vi "Checksum.vi"(0 "VISA resource name":refnum<visa-resource-name>, 5 "Command Frame Array":i16[](array[numeric]), 11 "error in (no error)":errorcluster) -> (4 "VISA resource name out":refnum<visa-resource-name>, 6 "Output String":string, 8 "Output Array":i16[](array[numeric]), 10 "Checksum":i16, 15 "error out":errorcluster)   [LabVIEW 2019, in "BK Precision 178XB Series.lvlib"]
doc: "This SubVI calculates the checksum of all bytes in the <b>Command frame array</b>, which is an array of 26 bytes. The checksum value takes the sum of the first 25 bytes in the array, and places the result into the last byte (26th byte). The <b>Output array</b> will be the resulting 26 byte array with the checksum value as the element of the last byte. <b>Output string</b> is the converted string from <b>Output array</b>.\n\nThe <b>Checksum</b> output will give the value of the checksum only."
uses:
  BK Precision 178XB Series.lvlib
panel:
  # "(c) 2009 B&K PRECISION CORPORATION.  ALL RIGHTS RESERVED."
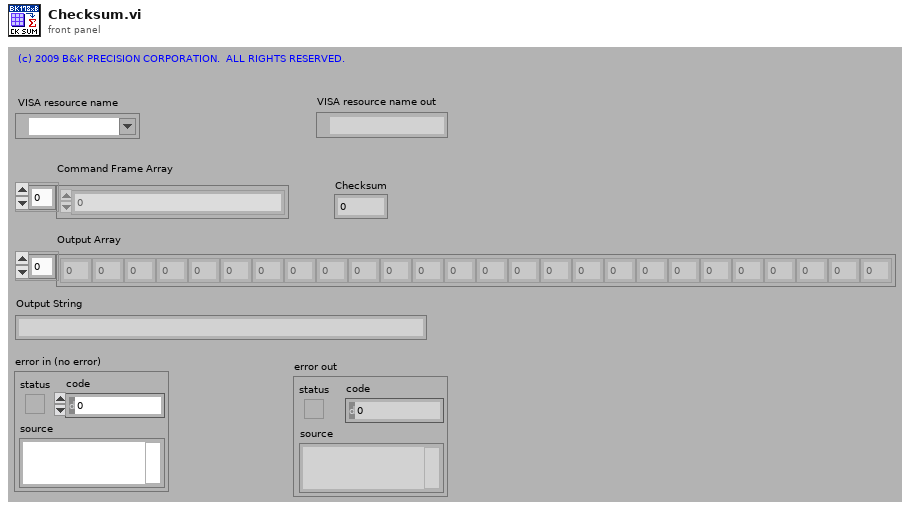
[diagram p1: front panel]
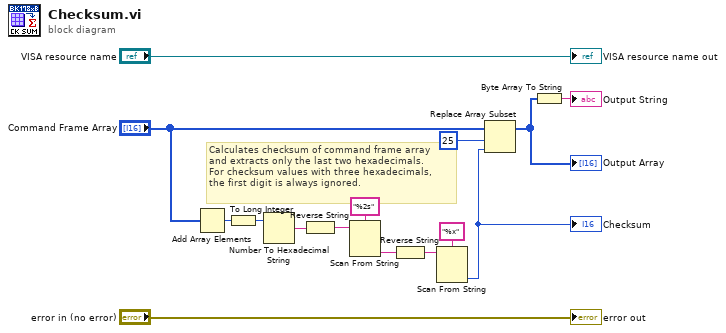
[diagram p0: block diagram]
diagram:
  # "Calculates checksum of command frame array\nand extracts only the last two hexadecimals. \nFor checksum values with three hexadecimals,\nthe first digit is always ignored."
  n1 = Add Array Elements(numeric array="Command Frame Array") -> (sum=w12:i16)
  n2 = To Long Integer(number=w12) -> (32bit integer=w14:i32)
  n3 = Number To Hexadecimal String(2:w14) -> (0:w8:string)  [unwired: 1 in]
  n4 = Reverse String(1:w8) -> (0:w15:string)
  n5 = Scan From String(format string="%2s", input string=w15) -> (output 1=w11:string)  [unwired: 3 in, 3 out]
  n6 = Reverse String(1:w11) -> (0:w10:string)
  n7 = Scan From String(format string="%x", input string=w10) -> (output 1=w4:i16)  [unwired: 3 in, 3 out]
  "Checksum" <- w4
  n8 = Replace Array Subset(array="Command Frame Array", new element=w4, index=25) -> (w2:i16[])
  "Output Array" <- w2
  n9 = Byte Array To String(unsigned byte array=w2) -> (string=→"Output String":string)
  "error out" <- "error in (no error)"
  "VISA resource name out" <- "VISA resource name"
